vi "sub parse frame c.vi"(8 "error in (no error)":errorcluster, 11 "<c> String":string="   <o kind 1 x 46 y 75 action 70 oid 204 o>") -> (0 "error out":errorcluster, 3 "<c> data":T1)   [LabVIEW 2018, in "Frame Analizer.lvclass"]
uses:
  Frame Analizer.lvclass
  frame c data.ctl
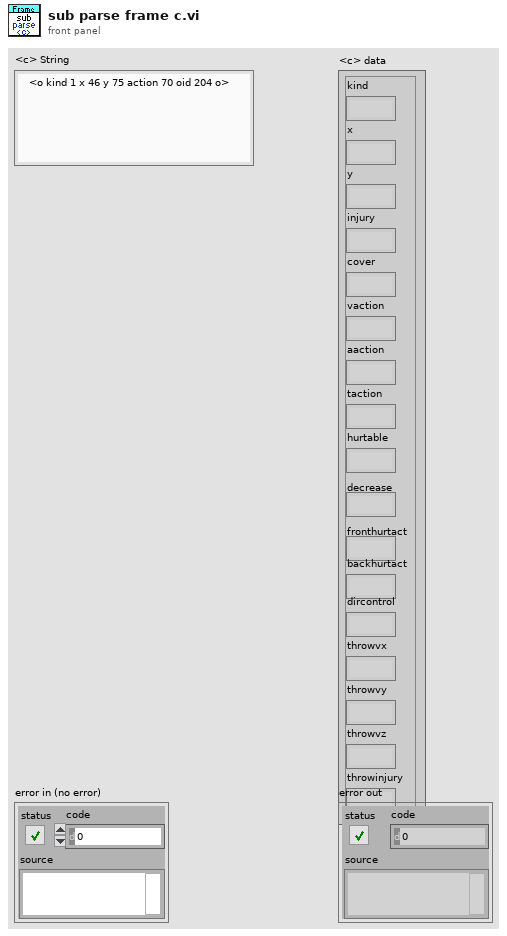
[diagram p1: front panel]
types:
  T1 = typedef "Frame Analizer.lvclass/frame c data.ctl" = cluster{"kind":string, "x":string, "y":string, "injury":string, "cover":string, "vaction":string, "aaction":string, "taction":string, "hurtable":string, "decrease":string, "fronthurtact":string, "backhurtact":string, "dircontrol":string, "throwvx":string, "throwvy":string, "throwvz":string, "throwinjury":string}
  T2 = cluster{"[0]":string, "[1]":string, "[2]":string, "[3]":string, "[4]":string, "[5]":string, "[6]":string, "[7]":string, "[8]":string, "[9]":string, "[10]":string, "[11]":string, "[12]":string, "[13]":string, "[14]":string, "[15]":string, "[16]":string}
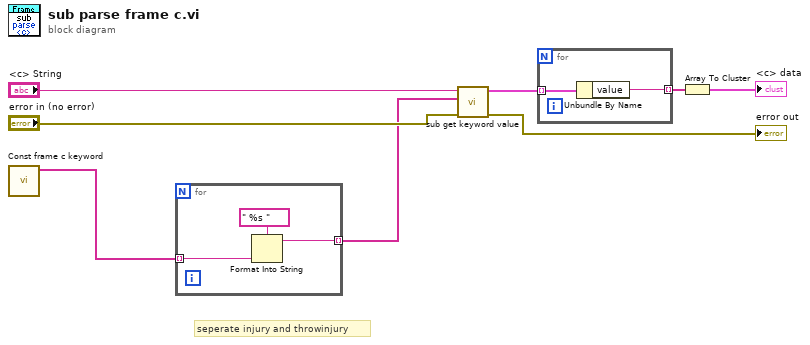
[diagram p0: block diagram]
diagram:
  # "seperate injury and throwinjury"
  n1 = call "Const frame c keyword.vi"() -> ("Const frame c keyword"=w2:string[])  [unwired: 11 in]
  n2 = for {
    tunnel: w2 -> [w11] mode=indexing
    tunnel: [w9] -> w1 mode=indexing
    n3 = Format Into String(format string=" %s ", w11) -> (resulting string=w9:string)  [unwired: 2 in, 1 out]
  }
  n4 = call "sub get keyword value.vi"("error in"="error in (no error)", "keyword"=w1, "string"="<c> String") -> ("error out"=→"error out":errorcluster, "matched pairs (all)"=w5:cluster{"keyword":string, "value":string}[])  [unwired: 5 in, 2 out]
  n5 = for {
    tunnel: w5 -> [w13] mode=indexing
    tunnel: [w12] -> w4 mode=indexing
    n6 = Unbundle By Name(w13) -> ("value"=w12:string)
  }
  n7 = Array To Cluster(array=w4) -> (cluster=→"<c> data":T2)
